vi "8 and 4 pulses TX 16spc.vi"(7 "reset system clock":bool, 8 "referenses 2":T1={"clock x2"="IO Socket\\Data Clock 2x", "Memory In"="pulse on memory", "Memory In 2"="pulse on memory", "Memory In 3"="pulse on memory", "Memory In 4"="pulse on memory"}, 9 "IQ_run":bool=TRUE, 10 "PDW input Valid":bool, 11 "array PDW":u64[](array[numeric])=[0, 0, 0, 0]) -> (1 "pulse TX status":T2, 2 "output valid":bool, 3 "IQ out":T3[](array[typedef]), 4 "ready for input":bool)   [LabVIEW 2021]
uses:
  <instrlib>/_niInstr/DSP/v1/Shared/Public/IQ Data.ctl
  pulse_tx_vis/CTL/mode_type.ctl
  <instrlib>/_niInstr/Basic Elements/v1/FPGA/Private/Count Up U64.vi
  <instrlib>/_niInstr/Basic Elements/v1/FPGA/Private/Count Up U32.vi
  <instrlib>/_niInstr/Basic Elements/v1/FPGA/niInstr Basic Elements v1 FPGA.lvlib
  <instrlib>/_niInstr/DSP/v1/Shared/niInstr DSP v1 Shared.lvlib
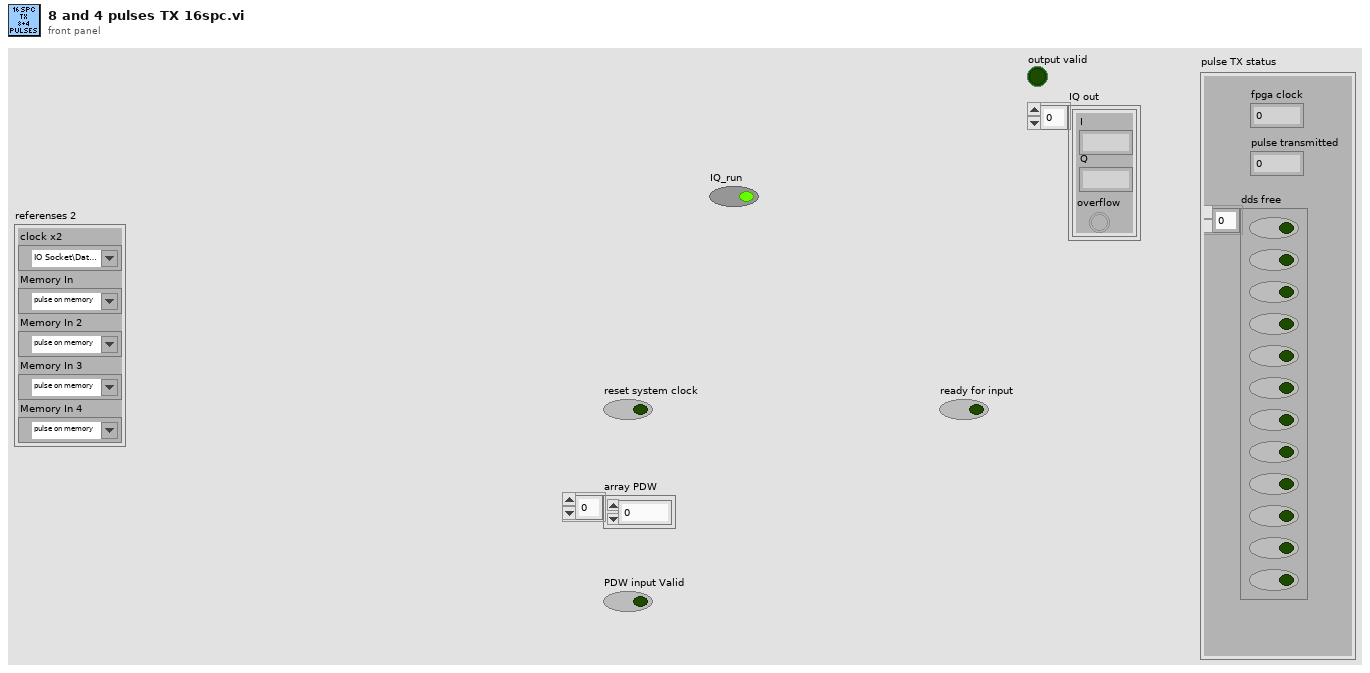
[diagram p1: front panel]
types:
  T1 = cluster{"clock x2":refnum<k21>, "Memory In":refnum<k21>, "Memory In 2":refnum<k21>, "Memory In 3":refnum<k21>, "Memory In 4":refnum<k21>}
  T2 = cluster{"fpga clock":u64, "pulse transmitted":u32, "dds free":bool[]}
  T3 = typedef "niInstr DSP v1 Shared.lvlib/IQ Data.ctl" = cluster{"I":fxp<+/-,18,1>, "Q":fxp<+/-,18,1>, "overflow":bool}
  T4 = typedef "mode_type.ctl" = enum8{"CW", "from memory 1", "NC - cw", "LFM", "BPSK", "QPSK"}
  T5 = typedef "pdw.ctl" = cluster{"PW":u32, "frequency shift":fxp<+/-,48,0>, "amp":fxp<+/-,18,1>, "mode type":T4, "mode depth":u32, "mode filter":u8, "phase shift":fxp<+/-,16,1>, "pulse shape filter":u8}
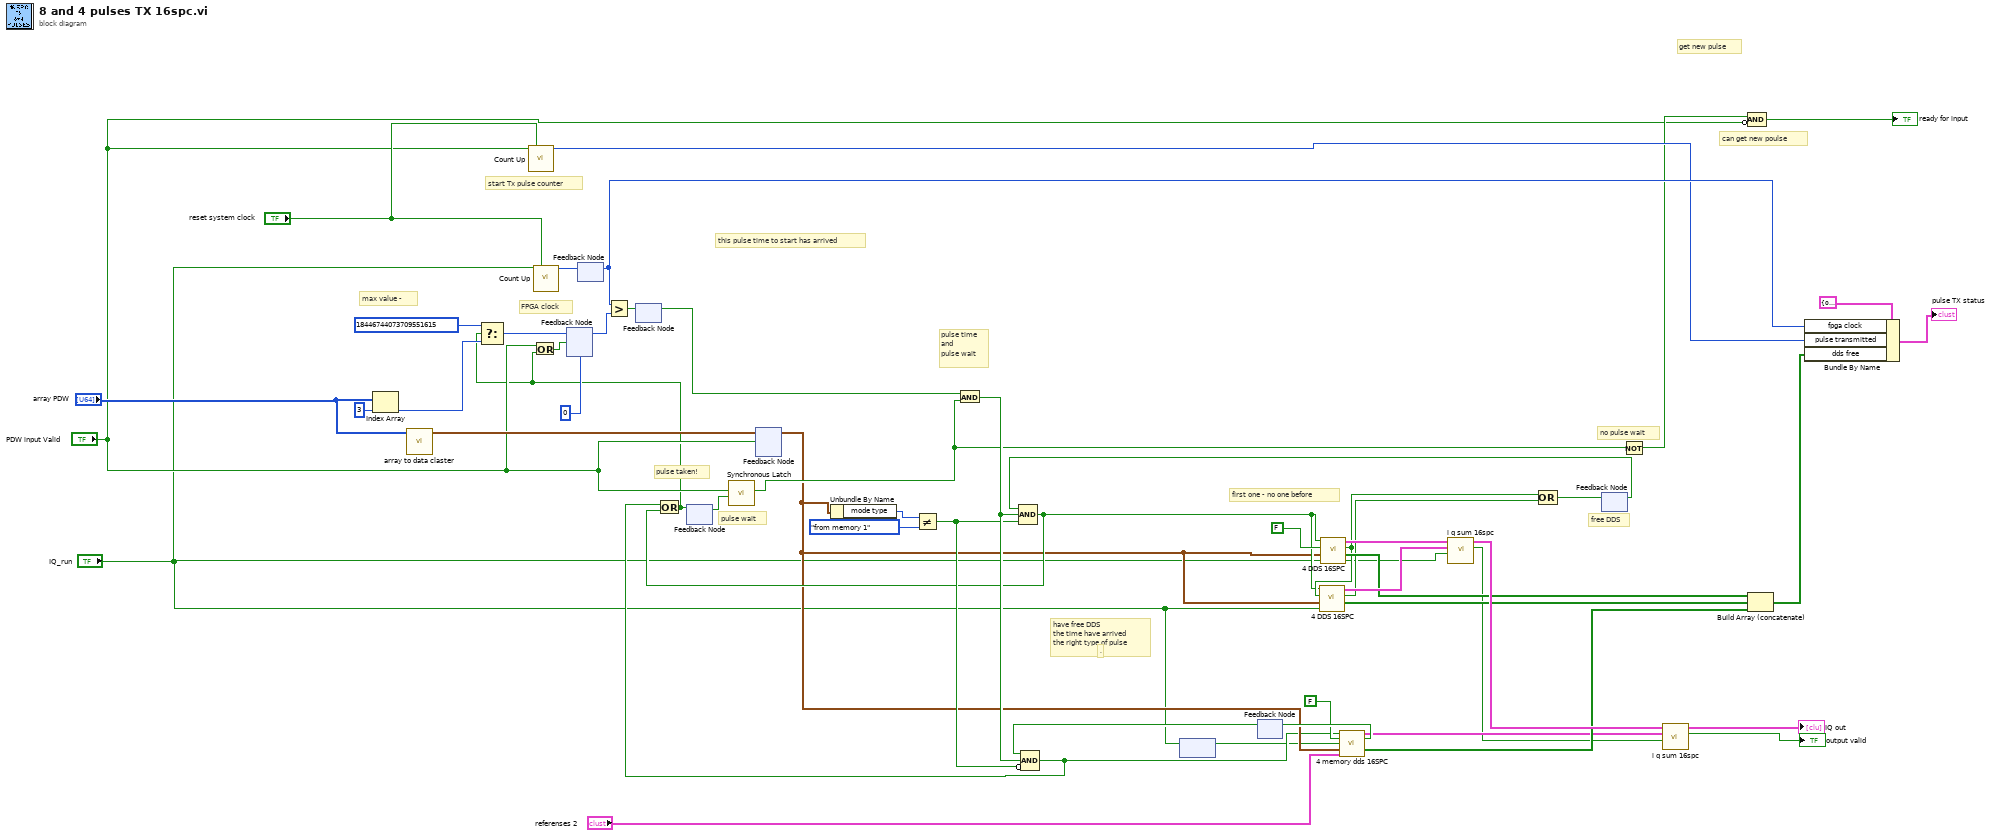
[diagram p0: block diagram]
diagram:
  # "have free DDS\nthe time have arrived\nthe right type of pulse"
  # "."
  # "pulse taken!"
  # "start Tx pulse counter"
  # "FPGA clock"
  # "this pulse time to start has arrived"
  # "first one - no one before"
  # "max value -"
  # "pulse time\nand\npulse wait"
  # "get new pulse"
  # "pulse wait"
  # "can get new poulse"
  # "no pulse wait"
  # "free DDS"
  n1 = Index Array(array="array PDW", index=3) -> (element=w49:u64)
  n2 = call "array to data claster.vi"("Array"="array PDW") -> ("Cluster"=w27:T5)  [unwired: 10 in]
  n3 = call-poly <instrlib>:"Count Up.vi"("increment"="PDW input Valid", "reset"="reset system clock") -> ("count out"=w29:u32)  [unwired: 13 in]
  n4 = call-poly <instrlib>:"Count Up.vi"("increment"="IQ_run", "reset"="reset system clock") -> ("count out"=w45:u64)  [unwired: 13 in]
  n5 = feedback #1(u64 0 ("U64")) -> (w38:u64)
  n6 = feedback #2() -> (w30:u64)  [unwired: 1 in]
  n7 = feedback-in #2(w45) -> ()
  n8 = Greater?(x=w30, y=w38) -> (0:w52:bool)
  n9 = feedback #3() -> (w53:bool)  [unwired: 1 in]
  n10 = feedback-in #3(w52) -> ()
  n11 = feedback #4() -> (w15:bool)  [unwired: 1 in]
  n12 = call <instrlib>:"Synchronous Latch.vi"("clear"=w15, "set"="PDW input Valid") -> ("out"=w16:bool)  [unwired: 9 in]
  n13 = feedback #5() -> (w11:T5)  [unwired: 1 in]
  n14 = feedback-in #5(w27, "PDW input Valid") -> ()
  n15 = Unbundle By Name(w11) -> ("mode type"=w26:T4)
  n16 = Not Equal?(x=w26, y=mode_type."from memory 1") -> (x != y?=w21:bool)
  n17 = And(x=w53, y=w16) -> (x .and. y?=w22:bool)
  n18 = feedback #6() -> (w3:bool)  [unwired: 1 in]
  n19 = feedback-in #6("IQ_run") -> ()
  n20 = feedback #7() -> (w13:bool)  [unwired: 1 in]
  n21 = Compound Arithmetic op=AND(w13, w22, invert w21) -> (w9:bool)
  n22 = call "4 memory dds 16SPC.vi"("new PDW in"=w9, "free DDS before me?"=FALSE, "run"=w3, "pdw in"=w11, "referenses"="referenses 2") -> ("IQ out"=w5:T3[], "have free DDS"=w12:bool, "state of every DDS"=w7:bool[])  [unwired: 7 in, 1 out]
  n23 = feedback-in #7(w12) -> ()
  n24 = feedback #8() -> (w18:bool)  [unwired: 1 in]
  n25 = Compound Arithmetic op=AND(w18, w22, w21) -> (w14:bool)
  n26 = Or(x=w9, y=w14) -> (x .or. y?=w1:bool)
  n27 = Select(t=u64 18446744073709551615, s=w1, f=w49) -> (s? t:f=w41:u64)
  n28 = Or(x="PDW input Valid", y=w1) -> (x .or. y?=w42:bool)
  n29 = feedback-in #1(w41, w42) -> ()
  n30 = feedback-in #4(w1) -> ()
  n31 = call "4 DDS 16SPC.vi"("input valid"="IQ_run", "pdw in"=w11, "free DDS before me?"=FALSE, "new PDW in"=w14) -> ("output valid"=w6:bool, "state of every DDS"=w37:bool[], "have free DDS"=w33:bool, "IQ out"=w35:T3[])  [unwired: 4 in]
  n32 = call "4 DDS 16SPC.vi"("input valid"="IQ_run", "pdw in"=w11, "free DDS before me?"=w33, "new PDW in"=w14) -> ("state of every DDS"=w36:bool[], "have free DDS"=w34:bool, "IQ out"=w48:T3[])  [unwired: 4 in, 1 out]
  n33 = call "i q sum 16spc.vi"("input valid"=w6, "IQ in 2"=w48, "IQ in"=w35) -> ("output valid"=w2:bool, "IQ out"=w46:T3[])  [unwired: 7 in]
  n34 = Compound Arithmetic op=OR(w33, w34) -> (w19:bool)
  n35 = feedback-in #8(w19) -> ()
  n36 = Not(x=w16) -> (.not. x?=w20:bool)
  n37 = call "i q sum 16spc.vi"("input valid"=w2, "IQ in 2"=w5, "IQ in"=w46) -> ("output valid"=→"output valid":bool, "IQ out"=→"IQ out":T3[])  [unwired: 7 in]
  n38 = Compound Arithmetic op=AND(w20, invert "PDW input Valid") -> (→"ready for input":bool)
  n39 = Build Array (concatenate)(w37, w36, w7) -> (w28:bool[])
  n40 = Bundle By Name(cluster=T2 {"fpga clock"=0, "pulse transmitted"=0, "dds free"=[FALSE, FALSE, FALSE, FALSE, FALSE, FALSE, FALSE, FALSE, FALSE, FALSE, FALSE, FALSE]} ("pulse TX status"), "fpga clock"=w30, "pulse transmitted"=w29, "dds free"=w28) -> (→"pulse TX status":T2)
